vi "Set cursor snap to plot.vi"(9 "Data In":T1, 11 "Waveform Graph in":T6) -> (3 "WaveformGraph out":T6)   [LabVIEW 2017, in "XGrapher.xctl"]
uses:
  XGrapher.xctl
  Typedefs/Xctrl-Waveform graph ref.ctl
  Data 1.ctl
  Typedefs/Xctrl-Data array.ctl
  Typedefs/Xcrtl-Data format definition.ctl
  Typedefs/Xctl-XY data type definition.ctl
  Typedefs/Xctrl-ROI type enum.ctl
panel:
  out "Selected POI index":u16
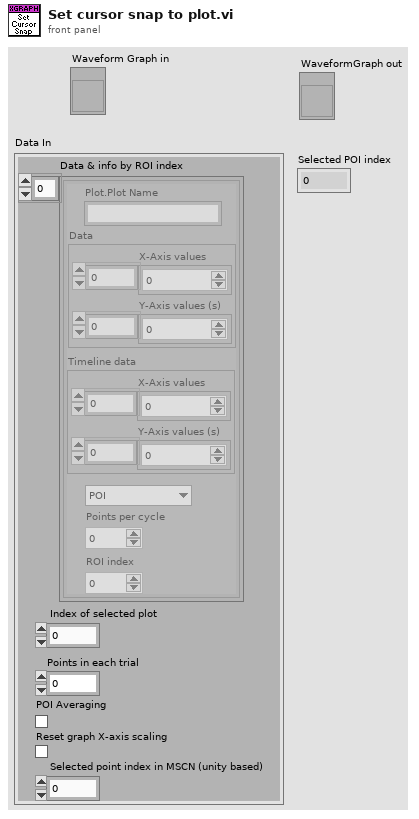
[diagram p1: front panel]
types:
  T1 = typedef "XGrapher.xctl/Data 1.ctl" = cluster{"Data & info by ROI index":T2, "Index of selected plot":u16, "Points in each trial":i32, "POI Averaging":bool, "Reset graph X-axis scaling":bool, "Selected point index in MSCN (unity based)":u16}
  T2 = typedef "Xctrl-Data array.ctl" = T3[]
  T3 = typedef "XGrapher.xctl/Xcrtl-Data format definition.ctl" = cluster{"Plot.Plot Name":string, "Data":T4, "Timeline data":T4, "Type":T5, "Points per cycle":u16, "ROI index":u16}
  T4 = typedef "XGrapher.xctl/Xctl-XY data type definition.ctl" = cluster{"X-Axis values":sgl[], "Y-Axis values (s)":sgl[]}
  T5 = typedef "Xctrl-ROI type enum.ctl" = enum16{"POI", "Mini-scan", "Group"}
  T6 = typedef "XGrapher.xctl/Xctrl-Waveform graph ref.ctl" = refnum<vi>
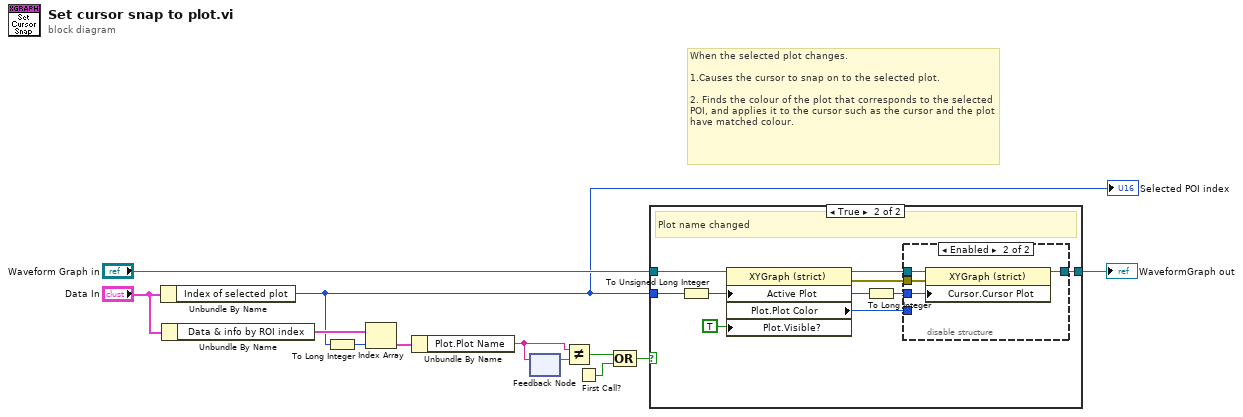
[diagram p0: block diagram]
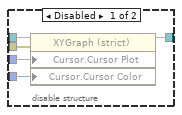
[diagram p3: hidden frame]
diagram:
  # "When the selected plot changes.\n\n1.Causes the cursor to snap on to the selected plot.\n\n2. Finds the colour of the plot that corresponds to the selected POI, and applies it to the cursor such as the cursor and the plot have matched colour."
  n1 = Unbundle By Name("Data In") -> ("Index of selected plot"=w1:u16)
  "Selected POI index" <- w1
  n2 = Unbundle By Name("Data In") -> ("Data & info by ROI index"=w6:T2)
  n3 = To Long Integer(number=w1) -> (32bit integer=w5:i32)
  n4 = Index Array(array=w6, index=w5) -> (element=w3:T3)
  n5 = Unbundle By Name(w3) -> ("Plot.Plot Name"=w2:string)
  n6 = feedback-in #1(w2) -> ()
  n7 = feedback #1() -> (w10:string)  [unwired: 1 in]
  n8 = Not Equal?(x=w2, y=w10) -> (x != y?=w9:bool)
  n9 = First Call?() -> (First Call?: T/F=w7:bool)
  n10 = Compound Arithmetic op=OR(w9, w7) -> (w8:bool)
  n11 = case shown="True" w8 {
    tunnel: [w13 w22] -> w12
    tunnel: "Waveform Graph in" -> [w13 w16]
    tunnel: w1 -> [_ w14]
    frame False {
    }
    frame True {
      # "Plot name changed"
      n12 = To Unsigned Long Integer(number=w14) -> (unsigned 32bit integer=w20:u32)
      n13 = property on="Get Plot's Color" class="XYGraph (strict)"(reference=w16, "Active Plot"=w20, "Plot.Visible?"=TRUE ("Plot.Visible")) -> (reference out=w17:T6, error out=w18:errorcluster, "Plot.Plot Color"=w19:u32)  [unwired: 1 in]
      n14 = To Long Integer(number=w20) -> (32bit integer=w21:i32)
      n15 = disable-structure shown="Enabled" {
        disable-tunnel: [w27 w31] -> w22
        disable-tunnel: w21 -> [w26 w30]
        disable-tunnel: w19 -> [w25 _]
        disable-tunnel: w18 -> [w24 w29]
        disable-tunnel: w17 -> [w23 w28]
        frame Disabled {
          n16 = property on="Get Plot's Color" class="XYGraph (strict)"(reference=w23, error in=w24, "Cursor.Cursor Plot"=w26, "Cursor.Cursor Color"=w25) -> (reference out=w27:T6)  [unwired: 1 out]
        }
        frame Enabled {
          n17 = property on="Get Plot's Color" class="XYGraph (strict)"(reference=w28, error in=w29, "Cursor.Cursor Plot"=w30) -> (reference out=w31:T6)  [unwired: 1 out]
        }
      }
    }
  }
  "WaveformGraph out" <- w12
